vi "ReadIniFile_LS1.vi"(8 "Error in":errorcluster) -> (0 "Error out":errorcluster, 1 "Experiment":path=path "C:/Données/Run003", 2 "Session":i32, 3 "Répertoire initial":path=path "C:/Données/Run003", 4 "Interface":path=path "C:/Données/Run003", 5 "AllowSave":bool)   [LabVIEW 2010]
doc: "Ce VI ouvre le fichier Ini de L'enregistreur de température et lit les valeurs des différentes sections"
uses:
  <vilib>/Utility/config.llb/Read Key (I32).vi
  <vilib>/Utility/config.llb/Read Key (String).vi
  <vilib>/Utility/config.llb/Read Key (Boolean).vi
  <vilib>/Utility/config.llb/Write Key (I32).vi
  <vilib>/Utility/config.llb/Write Key (String).vi
  <vilib>/Utility/config.llb/NI_LVConfig.lvlib
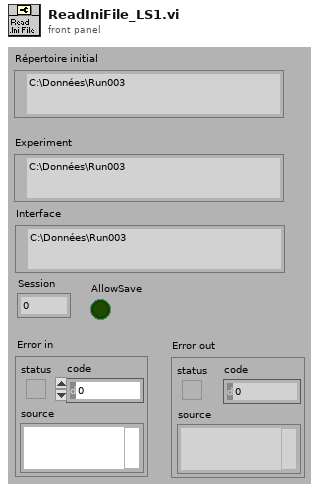
[diagram p1: front panel]
types:
  T1 = typedef "NI_LVConfig.lvlib/Config Data RefNum.ctl" = refnum<k1>
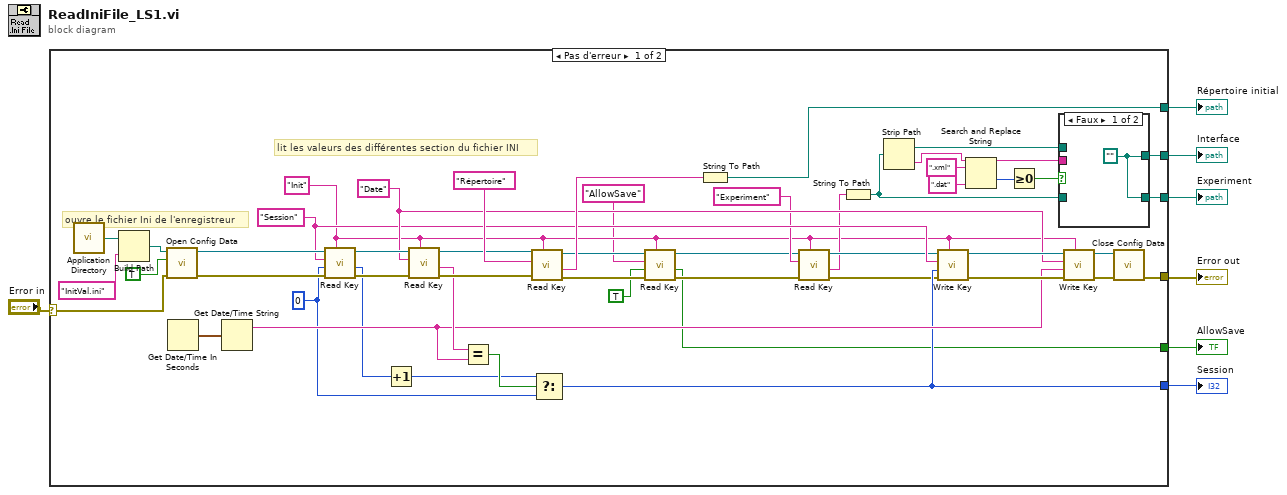
[diagram p0: block diagram]
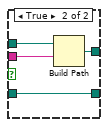
[diagram p2: hidden frame]
diagram:
  n1 = case shown="Pas d'erreur" "Error in" {
    selector: "Error in" -> [w55 w64]
    tunnel: [w50 w64] -> w7
    tunnel: [w52 _] -> w5
    tunnel: [w32 _] -> w4
    tunnel: [w18 _] -> w3
    tunnel: [w20 _] -> w2
    tunnel: [w8 _] -> w1
    frame No Error {
      w33 = 0
      w39 = "Date" ("key")
      w13 = "Init" ("section")
      w31 = "Session" ("key")
      # "lit les valeurs des différentes section du fichier INI"
      # "ouvre le fichier Ini de l'enregistreur"
      n2 = call <vilib>:"Application Directory.vi"() -> ("Application Directory"=w51:path)
      n3 = Build Path(base path=w51, name or relative path="InitVal.ini") -> (appended path=w56:path)
      n4 = call <vilib>:"Open Config Data.vi"("error in (no error)"=w55, "create file if necessary (T)"=TRUE ("create file if necessary? (T)"), "configuration file path"=w56) -> ("error out"=w48:errorcluster, "refnum"=w49:T1)  [unwired: 6 in, 1 out]
      n5 = Get Date/Time In Seconds() -> (seconds since 1Jan1904=w38:timestamp)
      n6 = Get Date/Time String(seconds (now)=w38) -> (date string=w36:string)  [unwired: 2 in, 1 out]
      n7 = call-poly <vilib>:"Read Key.vi"("section"=w13, "error in (no error)"=w48, "default value"=w33, "key"=w31, "refnum"=w49) -> ("error out"=w44:errorcluster, "value"=w35:i32, "refnum out"=w47:T1)  [unwired: 3 in, 1 out]
      n8 = Increment(x=w35) -> (x+1=w30:i32)
      n9 = call-poly <vilib>:"Read Key.vi"("section"=w13, "error in (no error)"=w44, "key"=w39, "refnum"=w47) -> ("error out"=w45:errorcluster, "value"=w37:string, "refnum out"=w46:T1)  [unwired: 4 in, 1 out]
      n10 = Equal?(x=w37, y=w36) -> (x = y?=w34:bool)
      n11 = call-poly <vilib>:"Read Key.vi"("section"=w13, "error in (no error)"=w45, "key"="Répertoire", "refnum"=w46) -> ("error out"=w15:errorcluster, "value"=w53:string, "refnum out"=w12:T1)  [unwired: 4 in, 1 out]
      n12 = Select(t=w30, s=w34, f=w33) -> (s? t:f=w32:i32)
      n13 = call-poly <vilib>:"Read Key.vi"("section"=w13, "error in (no error)"=w15, "default value"=TRUE, "key"="AllowSave", "refnum"=w12) -> ("error out"=w14:errorcluster, "value"=w8:bool, "refnum out"=w9:T1)  [unwired: 3 in, 1 out]
      n14 = String To Path(string=w53) -> (path=w52:path)
      n15 = call-poly <vilib>:"Read Key.vi"("section"=w13, "error in (no error)"=w14, "key"="Experiment", "refnum"=w9) -> ("error out"=w29:errorcluster, "value"=w26:string, "refnum out"=w27:T1)  [unwired: 4 in, 1 out]
      n16 = String To Path(string=w26) -> (path=w19:path)
      n17 = Strip Path(path=w19) -> (stripped path=w21:path, name=w24:string)
      n18 = call-poly <vilib>:"Write Key.vi"("section"=w13, "error in (no error)"=w29, "value"=w32, "key"=w31, "refnum"=w27) -> ("error out"=w43:errorcluster, "refnum out"=w40:T1)  [unwired: 4 in, 1 out]
      n19 = Search and Replace String(input string=w24, search string=".xml" ("chaîne recherchée"), replace string=".dat" ("chaîne de remplacement (\"\")")) -> (result string=w22:string, offset past replacement=w17:i32)  [unwired: 5 in, 2 out]
      n20 = Greater Or Equal To 0?(x=w17) -> (x >= 0?=w16:bool)
      n21 = case shown="Faux" w16 {
        tunnel: w22 -> [_ w63]
        tunnel: w21 -> [_ w62]
        tunnel: [w59 w61] -> w20
        tunnel: w19 -> [_ w60]
        tunnel: [w59 w60] -> w18
        frame False {
          w59 = path ""
        }
        frame True {
          n22 = Build Path(base path=w62, name or relative path=w63) -> (appended path=w61:path)
        }
      }
      n23 = call-poly <vilib>:"Write Key.vi"("section"=w13, "error in (no error)"=w43, "value"=w36, "key"=w39, "refnum"=w40) -> ("error out"=w42:errorcluster, "refnum out"=w41:T1)  [unwired: 4 in, 1 out]
      n24 = call <vilib>:"Close Config Data.vi"("error in (no error)"=w42, "refnum"=w41) -> ("error out"=w50:errorcluster)  [unwired: 8 in, 1 out]
    }
    frame Error {
    }
  }
  "Error out" <- w7
  "Répertoire initial" <- w5
  "Session" <- w4
  "Experiment" <- w3
  "Interface" <- w2
  "AllowSave" <- w1
